vi "DO-DI test MAX FPGA.vi"() -> ()   [LabVIEW 2014]
uses:
  <vilib>/rvi/Emulation/niFpgaGetClockAttributes.vi
  <vilib>/rvi/Emulation/niFpgaSctlEmulationGetInTimedLoop.vi
  <vilib>/rvi/Emulation/niFpgaEmulationReportErrorSimple.vi
  <vilib>/rvi/eio/common/nirviEmuTemplateMethod_errors.vi
  <vilib>/rvi/Emulation/niFpgaCriticalErrorInLSC.vi
  <vilib>/eio/EIONode/EIONode.xnode
panel:
  out "eSTOP":bool
  out "CO_GLD":bool
  out "HC_GLD":bool
  out "NO_GLD":bool
  out "Air_PS":bool
  out "NO_PS":bool
  out "AirBal_PS":bool
  out "HC_PS":bool
  out "CO_PS":bool
  out "N_PS":bool
  out "CO2_PS":bool
  out "Ext gas meas D":bool
  out "Temp_SW1":bool
  out "Door1 open":bool
  out "Door2 open":bool
  out "Extractor Fan":bool
  out "Ext gas meas U":bool
  out "Mod1_01":bool
  out "Mod1_02":bool
  out "SO2_GLD":bool
  out "Mod1 07":bool
  out "Mod1 08":bool
  out "SO2_PS":bool
  out "H2O_PS":bool
  out "Mod1_18":bool
  out "Mod1_19":bool
  out "Temp_SW2":bool
  out "Mod1_22":bool
  out "Mod1_28":bool
  out "Mod1_29":bool
  out "Mod1_30":bool
  out "Mod1_31":bool
  in  "CUT-Off_2":bool
  in  "CUT-Off_1":bool
  in  "OEM_Alarm/E_SV-4":bool
  in  "NOx_Can/E_SV-3":bool
  in  "Pump/E_SV-2":bool
  in  "Door":bool
  in  "Extractor":bool
  in  "Inverter_On":bool
  in  "E_SV-1":bool
  in  "ISO7_SV":bool
  in  "ISO6_SV":bool
  in  "Vent2_ISO5_SV":bool
  in  "Vent1_ISO4_SV":bool
  in  "Buler-V_ISO3_SV":bool
  in  "Buler-B_ISO2_SV":bool
  in  "Buler-A_ISO1_SV":bool
  in  "Tank-PR_SV":bool
  in  "02_DO/DO14":bool
  in  "02_DO/DO13":bool
  in  "HC2_SV":bool
  in  "N2-P_SV":bool
  in  "Air2_SV":bool
  in  "HCBal_SV":bool
  in  "AirBal_SV":bool
  in  "H2O_SV":bool
  in  "N2_SV":bool
  in  "SO2_SV":bool
  in  "CO2_SV":bool
  in  "NO_SV":bool
  in  "Air1_SV":bool
  in  "HC1_SV":bool
  in  "CO_SV":bool
  in  "stop":bool
  # "Test App Digital Out and Digital In"
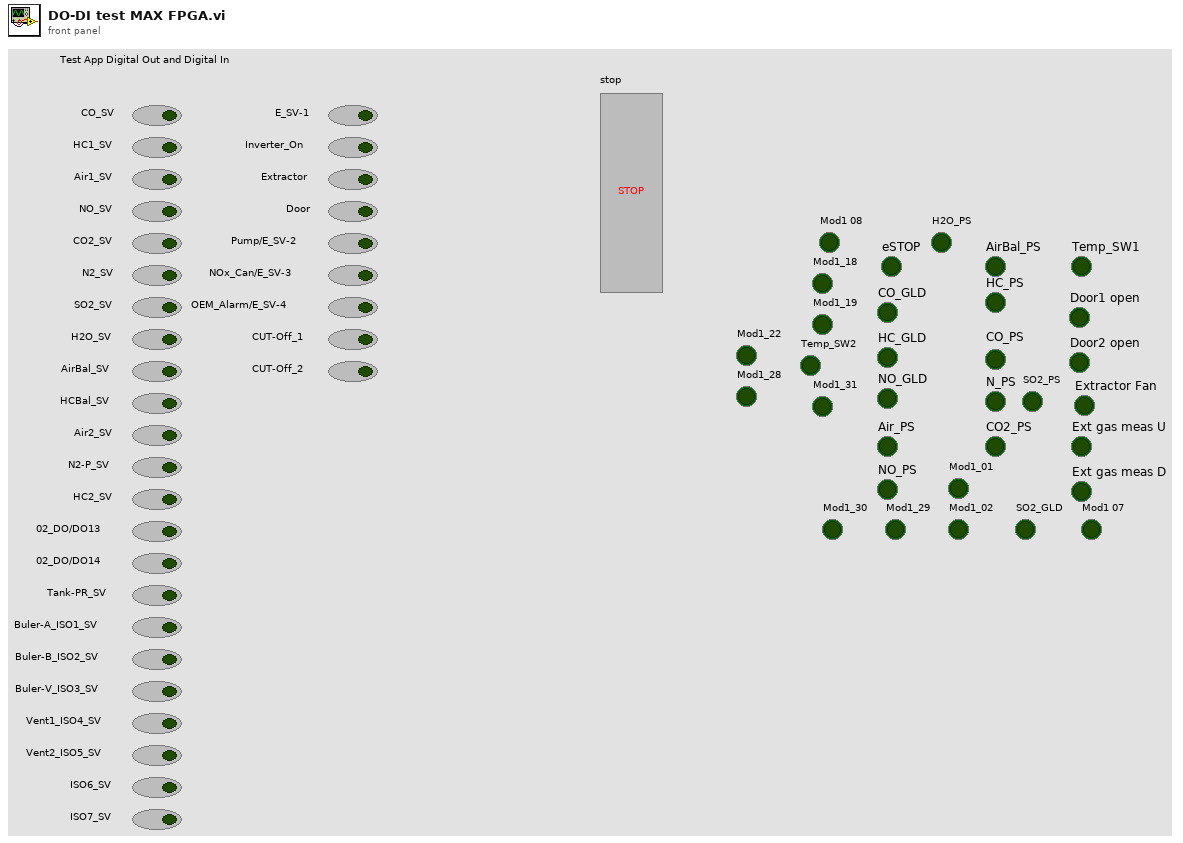
[diagram p1: front panel]
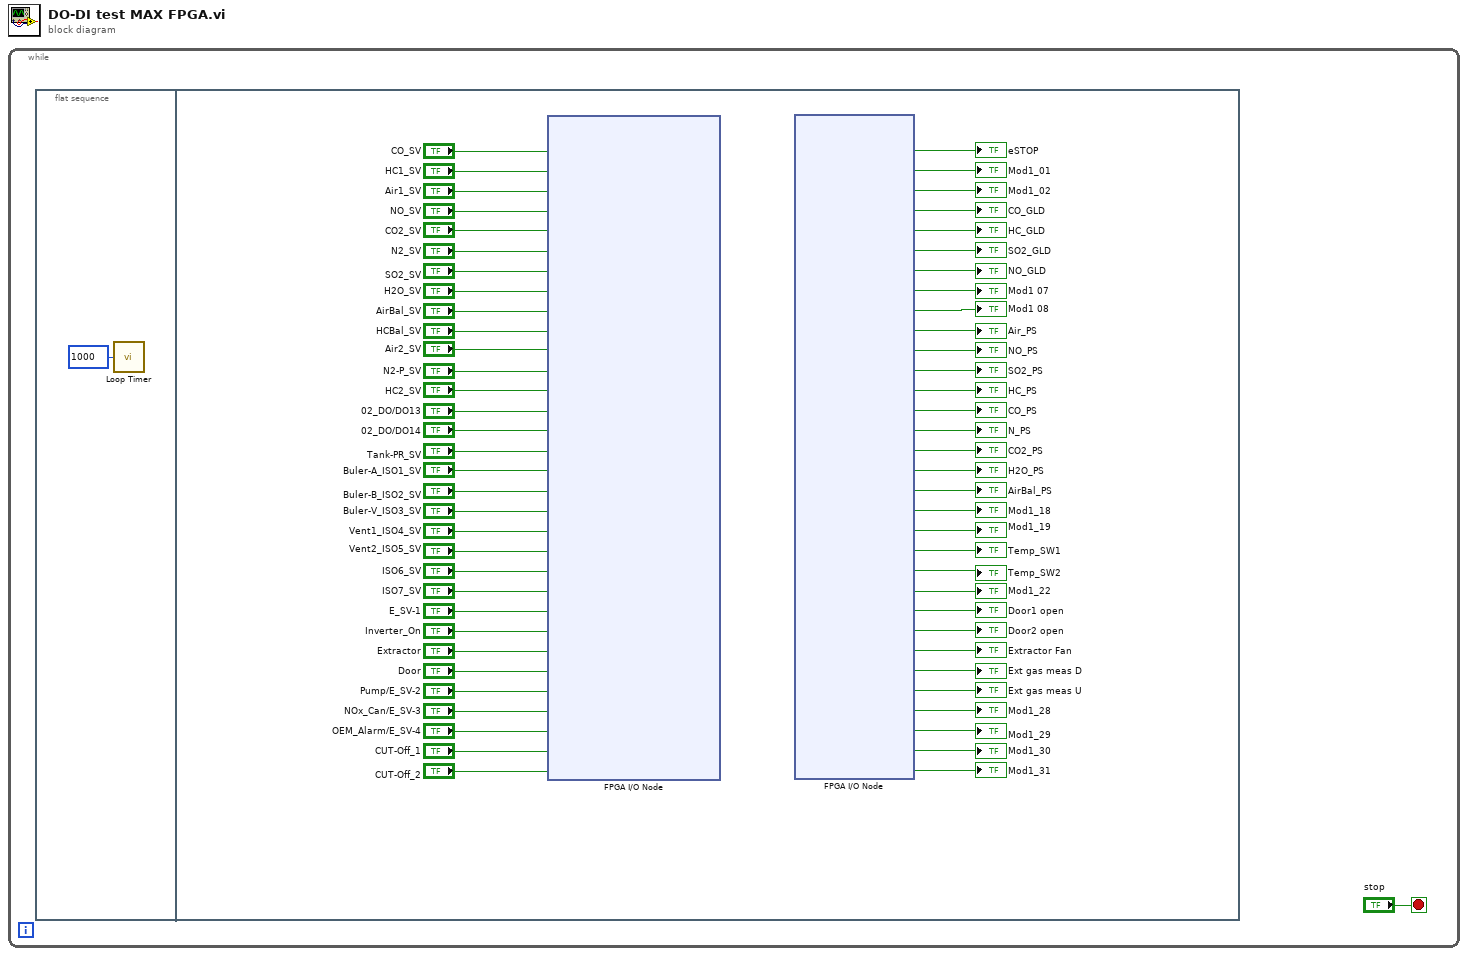
[diagram p0: block diagram]
diagram:
  n1 = while {
    stop <- "stop" stop-if-true
    n2 = flat-sequence {
      frame #0 {
        n3 = call "Loop Timer"("Count(mSec)"=u32 1000) -> ()  [unwired: 1 out]
      }
      frame #1 {
        n4 = xnode "FPGA I/O Node"("CO_SV"="CO_SV", "HC1_SV"="HC1_SV", "Air1_SV"="Air1_SV", "NO_SV"="NO_SV", "CO2_SV"="CO2_SV", "N2_SV"="N2_SV", "SO2_SV"="SO2_SV", "H2O_SV"="H2O_SV", "AirBal_SV"="AirBal_SV", "HCBal_SV"="HCBal_SV", "Air2_SV"="Air2_SV", "N2-P_SV"="N2-P_SV", "HC2_SV"="HC2_SV", "02_DO/DO13"="02_DO/DO13", "02_DO/DO14"="02_DO/DO14", "Tank-PR_SV"="Tank-PR_SV", "Buler-A_ISO1_SV"="Buler-A_ISO1_SV", "Buler-B_ISO2_SV"="Buler-B_ISO2_SV", "Buler-V_ISO3_SV"="Buler-V_ISO3_SV", "Vent1_ISO4_SV"="Vent1_ISO4_SV", "Vent2_ISO5_SV"="Vent2_ISO5_SV", "ISO6_SV"="ISO6_SV", "ISO7_SV"="ISO7_SV", "E_SV-1"="E_SV-1", "Inverter_On"="Inverter_On", "Extractor"="Extractor", "Door"="Door", "Pump/E_SV-2"="Pump/E_SV-2", "NOx_Can/E_SV-3"="NOx_Can/E_SV-3", "OEM_Alarm/E_SV-4"="OEM_Alarm/E_SV-4", "CUT-Off_1"="CUT-Off_1", "CUT-Off_2"="CUT-Off_2") -> ()  [unwired: 32 in, 32 out]
        n5 = xnode "FPGA I/O Node"() -> ("eStop"=→"eSTOP":bool, "Mod1_01"=→"Mod1_01":bool, "Mod1_02"=→"Mod1_02":bool, "CO_GLD"=→"CO_GLD":bool, "HC_GLD"=→"HC_GLD":bool, "SO2_GLD"=→"SO2_GLD":bool, "NO_GLD"=→"NO_GLD":bool, "Mod1 07"=→"Mod1 07":bool, "Mod1 08"=→"Mod1 08":bool, "Air_PS"=→"Air_PS":bool, "NO_PS"=→"NO_PS":bool, "SO2_PS"=→"SO2_PS":bool, "HC_PS"=→"HC_PS":bool, "CO_PS"=→"CO_PS":bool, "N_PS"=→"N_PS":bool, "CO2_PS"=→"CO2_PS":bool, "H2O_PS"=→"H2O_PS":bool, "AirBal_PS"=→"AirBal_PS":bool, "Mod1_18"=→"Mod1_18":bool, "Mod1_19"=→"Mod1_19":bool, "Temp_SW1"=→"Temp_SW1":bool, "Temp_SW2"=→"Temp_SW2":bool, "Mod1_22"=→"Mod1_22":bool, "DR-1_Open"=→"Door1 open":bool, "DR-2_Open"=→"Door2 open":bool, "Fan_on"=→"Extractor Fan":bool, "EGMD"=→"Ext gas meas D":bool, "EGMU"=→"Ext gas meas U":bool, "Mod1_28"=→"Mod1_28":bool, "Mod1_29"=→"Mod1_29":bool, "Mod1_30"=→"Mod1_30":bool, "Mod1_31"=→"Mod1_31":bool)  [unwired: 32 in, 32 out]
      }
    }
  }
